vi "Help Query.vi"(8 "error in (no error)":errorcluster, 11 "VISA resource name":refnum<visa-resource-name>) -> (0 "error out":errorcluster, 2 "Help":string, 3 "VISA resource name out":refnum<visa-resource-name>)   [LabVIEW 2013, in "HadCon.lvlib"]
doc: "Queries the device help information."
uses:
  <instrlib>/HadCon/HadCon.lvlib
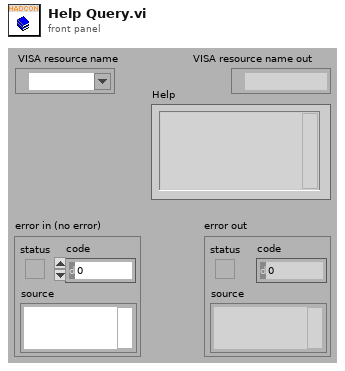
[diagram p1: front panel]
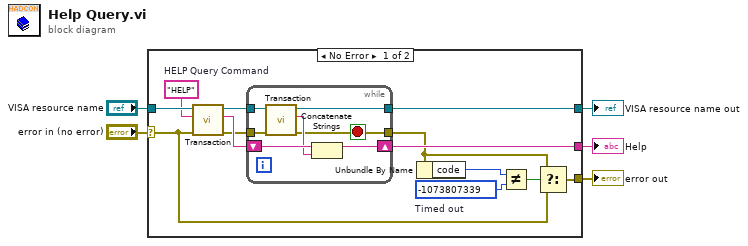
[diagram p0: block diagram]
diagram:
  n1 = case shown="No Error" "error in (no error)" {
    selector: "error in (no error)" -> [w11 w26]
    tunnel: [w9 w27] -> w5
    tunnel: "VISA resource name" -> [w18 w27]
    tunnel: [w8 w26] -> w3
    tunnel: [w16 _] -> w2
    frame No Error {
      w14 = -1073807339  # Timed out
      w10 = "HELP"  # HELP Query Command
      n2 = call <instrlib>:"Transaction.vi"("Error In"=w11, "Command"=w10, "VISA resource name"=w18) -> ("Error Out"=w6:errorcluster, "Response"=w17:string, "VISA resource name out"=w7:refnum<visa-resource-name>)  [unwired: 6 in]
      n3 = while {
        tunnel: w7 -> [w25]
        tunnel: w6 -> [w24]
        shift-right: [w21] -> w16
        shift-left: w17 -> [w23]
        tunnel: [w20] -> w9
        tunnel: [w19] -> w12
        stop <- w19 stop-if-true
        n4 = call <instrlib>:"Transaction.vi"("Error In"=w24, "VISA resource name"=w25) -> ("Error Out"=w19:errorcluster, "Response"=w22:string, "VISA resource name out"=w20:refnum<visa-resource-name>)  [unwired: 7 in]
        n5 = Concatenate Strings(w23, w22) -> (w21:string)
      }
      n6 = Unbundle By Name(w12) -> ("code"=w15:i32)
      n7 = Not Equal?(x=w15, y=w14) -> (x != y?=w13:bool)
      n8 = Select(t=w12, s=w13, f=w11) -> (s? t:f=w8:errorcluster)
    }
    frame Error {
    }
  }
  "VISA resource name out" <- w5
  "error out" <- w3
  "Help" <- w2
